vi "Chauvenet's criterion.vi"(0 "Input Data":dbl[](array[numeric]) format="%0.2f") -> (1 "Indices":i32[](array[numeric]), 2 "Outliers":dbl[](array[numeric]) format="%0.2f")   [LabVIEW 2017]
uses:
  <vilib>/gmath/statdist.llb/Normal PDF.vi
  <vilib>/Analysis/NI_AALBase.lvlib
  <vilib>/gmath/NI_Gmath.lvlib
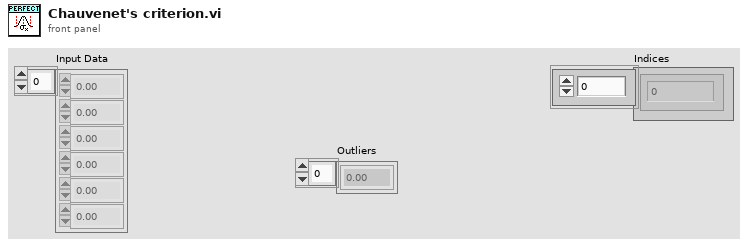
[diagram p1: front panel]
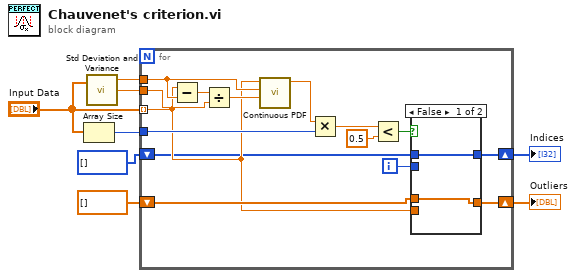
[diagram p0: block diagram]
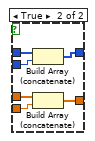
[diagram p2: hidden frame]
diagram:
  n1 = Array Size(array="Input Data") -> (size(s)=w5:i32)
  n2 = call <vilib>:"Std Deviation and Variance.vi"("X"="Input Data") -> ("mean"=w8:dbl, "standard deviation"=w7:dbl)  [unwired: 1 in, 1 out]
  n3 = for {
    tunnel: "Input Data" -> [w12] mode=indexing
    tunnel: w8 -> [w21]
    tunnel: w7 -> [w22]
    tunnel: w5 -> [w19]
    shift-right: [w15] -> w3
    shift-left: dbl[] [] -> [w14]
    shift-right: [w10] -> w1
    shift-left: i32[] [] -> [w9]
    i -> [w11]
    n4 = Subtract(x=w12, y=w21) -> (x-y=w23:dbl)
    n5 = Divide(x=w23, y=w22) -> (x/y=w13:dbl)
    n6 = call-poly <vilib>:"Continuous PDF.vi"("std"=w13, "mean"=w21, "x"=w12) -> ("pdf(x)"=w20:dbl)  [unwired: 7 in, 1 out]
    n7 = Multiply(x=w20, y=w19) -> (x*y=w18:dbl)
    n8 = Less?(x=w18, y=0.5) -> (x < y?=w16:bool)
    n9 = case shown="False" w16 {
      tunnel: w12 -> [_ w31]
      tunnel: [w25 w30] -> w15
      tunnel: w14 -> [w25 w29]
      tunnel: w11 -> [_ w28]
      tunnel: [w24 w27] -> w10
      tunnel: w9 -> [w24 w26]
      frame False {
      }
      frame True {
        n10 = Build Array (concatenate)(w26, w28) -> (w27:i32[])
        n11 = Build Array (concatenate)(w29, w31) -> (w30:dbl[])
      }
    }
  }
  "Outliers" <- w3
  "Indices" <- w1
